vi "T MeasurementTriton.vi"(1 "String":string="READ:DEV:T8:TEMP:SIG:TEMP\\r\\n", 7 "error out 2":errorcluster, 10 "VISA resource name 2":refnum<visa-resource-name>) -> (0 "error out":errorcluster, 2 "reading":string, 3 "VISA resource name":refnum<visa-resource-name>, 4 "Measuremet":dbl)   [LabVIEW 2021]
panel:
  out "General Settings:Timeout Value":u32
  out "TCP/IP Settings:Computer Hostname":string
  out "Message Based Settings:Termination Character Enable":bool
  out "Message Based Settings:Termination Character":u8
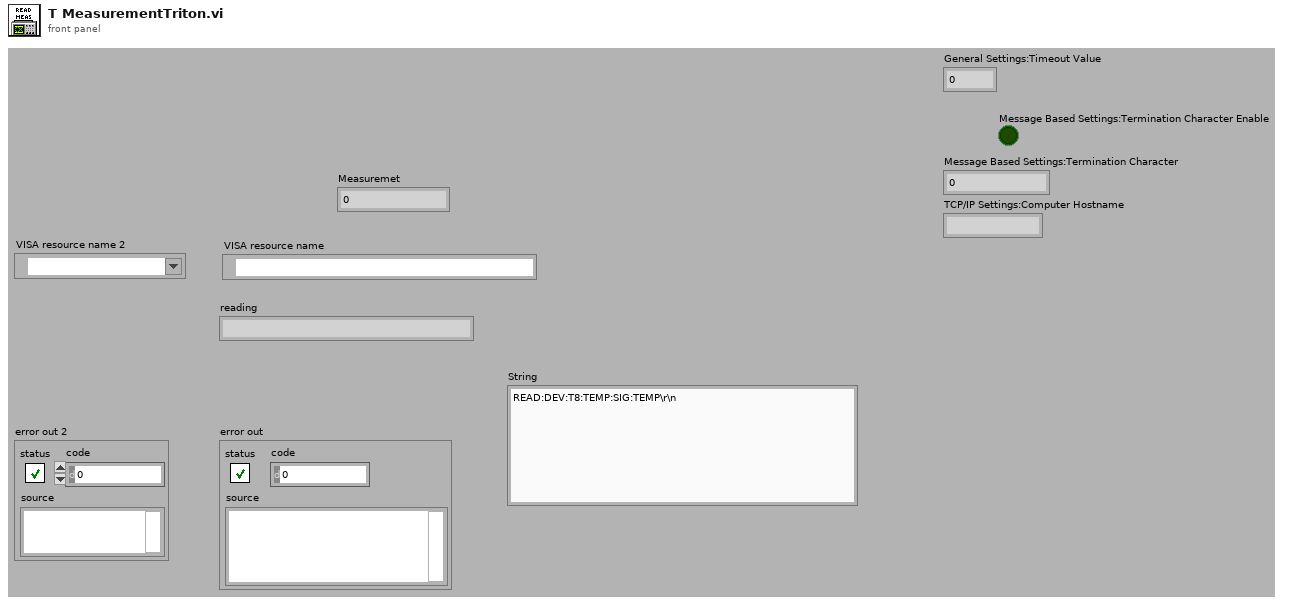
[diagram p1: front panel]
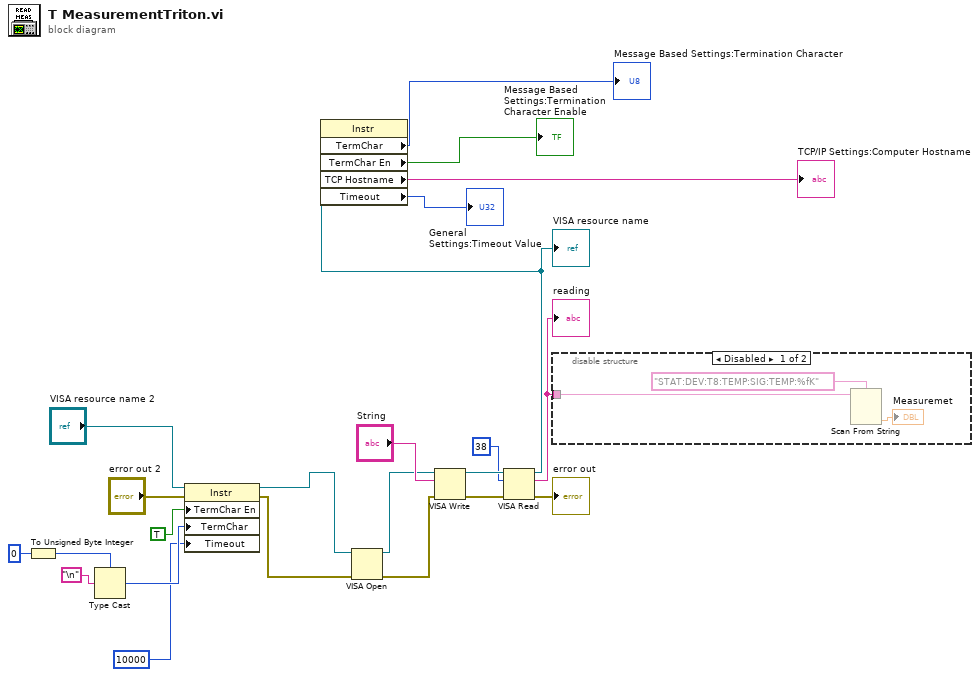
[diagram p0: block diagram]
diagram:
  n1 = To Unsigned Byte Integer(number=0) -> (unsigned 8bit integer=w10:u8)
  n2 = Type Cast(type=w10, x="\n") -> (*(type *) &x=w11:u8)
  n3 = property class="Instr"(reference="VISA resource name 2", error in="error out 2", "TermChar En"=TRUE ("Message Based Settings:Termination Character Enable"), "TermChar"=w11, "Timeout"=10000) -> (reference out=w8:refnum<visa-resource-name>, error out=w6:errorcluster)
  n4 = VISA Open(error in (no error)=w6, VISA resource name=w8) -> (VISA resource name=w7:refnum<visa-resource-name>, error out=w5:errorcluster)  [unwired: 3 in]
  n5 = VISA Write(VISA resource name=w7, write buffer="String", error in (no error)=w5) -> (VISA resource name out=w20:refnum<visa-resource-name>, error out=w16:errorcluster)  [unwired: 1 out]
  n6 = VISA Read(VISA resource name=w20, byte count=u32 38, error in (no error)=w16) -> (VISA resource name out=w4:refnum<visa-resource-name>, read buffer=w17:string, error out=→"error out":errorcluster)  [unwired: 1 out]
  "VISA resource name" <- w4
  "reading" <- w17
  n7 = property class="Instr"(reference=w4) -> ("TermChar"=→"Message Based Settings:Termination Character":u8, "TermChar En"=→"Message Based Settings:Termination Character Enable":bool, "TCP Hostname"=→"TCP/IP Settings:Computer Hostname":string, "Timeout"=→"General Settings:Timeout Value":u32)  [unwired: 1 in, 2 out]
  n8 = disable-structure shown="Disabled" {
    disable-tunnel: w17 -> [w26 _]
    frame Disabled {
      n9 = Scan From String(format string="STAT:DEV:T8:TEMP:SIG:TEMP:%fK", input string=w26) -> (output 1=→"Measuremet":dbl)  [unwired: 3 in, 3 out]
    }
    frame Enabled {
    }
  }
